vi "Check_for_Message_Parent.vi"(8 "error in (no error)":errorcluster, 11 "VI ref":refnum<vi>) -> (0 "error out":errorcluster, 1 "LVClassLibrary Refnum":refnum<vi>, 2 "Inherits from AF Message?":bool, 3 "VI ref out":refnum<vi>)   [LabVIEW 2015]
uses:
  <vilib>/ActorFramework/Message/Message.lvclass
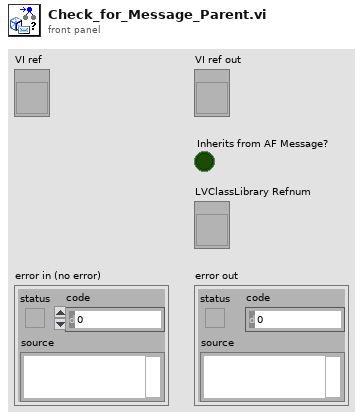
[diagram p1: front panel]
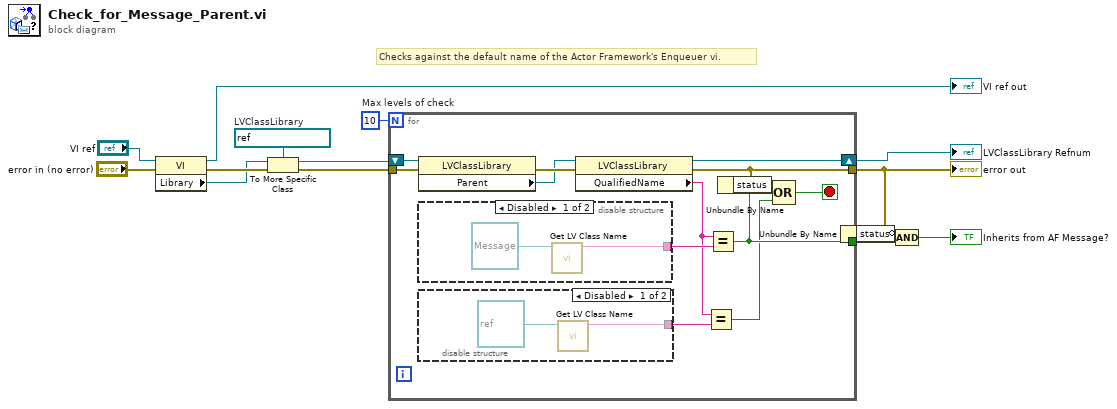
[diagram p0: block diagram]
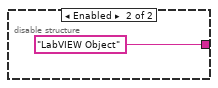
[diagram p2: hidden frame]
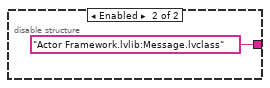
[diagram p3: hidden frame]
diagram:
  w13 = 10  # Max levels of check
  w14 = refnum<vi> refnum  # LVClassLibrary
  # "Checks against the default name of the Actor Framework's Enqueuer vi."
  n1 = property class="VI"(reference="VI ref", error in="error in (no error)") -> (reference out=→"VI ref out":refnum<vi>, error out=w9:errorcluster, "Library"=w8:refnum<vi>)
  n2 = To More Specific Class(target class=w14, reference=w8, error in=w9) -> (specific class reference=w6:refnum<vi>, error out=w7:errorcluster)
  n3 = for {
    N: w13 -> [_]
    tunnel: w7 -> [w26]
    tunnel: [w20] -> w12
    shift-right: [w22] -> w3
    shift-left: w6 -> [w27]
    tunnel: [w21] -> w5
    stop <- w16 stop-if-true
    n4 = property class="LVClassLibrary"(reference=w27, error in=w26) -> (error out=w24:errorcluster, "Parent"=w23:refnum<vi>)  [unwired: 1 out]
    n5 = disable-structure shown="Disabled" {
      disable-tunnel: [w31 "Actor Framework.lvlib:Message.lvclass" ("class name 2")] -> w25
      frame Disabled {
        n6 = call <vilib>:"Get LV Class Name.vi"("object"=refnum<class "Message.lvclass"> refnum ("Actor Framework:Message")) -> ("class name"=w31:string)  [unwired: 9 in, 1 out]
      }
      frame Enabled {
      }
    }
    n7 = disable-structure shown="Disabled" {
      disable-tunnel: [w28 "LabVIEW Object" ("class name 2")] -> w19
      frame Disabled {
        n8 = call <vilib>:"Get LV Class Name.vi"("object"=refnum<class> refnum) -> ("class name"=w28:string)  [unwired: 9 in, 1 out]
      }
      frame Enabled {
      }
    }
    n9 = property class="LVClassLibrary"(reference=w23, error in=w24) -> (reference out=w22:refnum<vi>, error out=w21:errorcluster, "QualifiedName"=w18:string)
    n10 = Equal?(x=w18, y=w19) -> (x = y?=w17:bool)
    n11 = Equal?(x=w18, y=w25) -> (x = y?=w20:bool)
    n12 = Unbundle By Name(w21) -> ("status"=w15:bool)
    n13 = Compound Arithmetic op=OR(w15, w20, w17) -> (w16:bool)
  }
  "error out" <- w5
  "LVClassLibrary Refnum" <- w3
  n14 = Unbundle By Name(w5) -> ("status"=w1:bool)
  n15 = Compound Arithmetic op=AND(invert w1, w12) -> (→"Inherits from AF Message?":bool)
